vi "Speed From FFT (FPGA).vi"() -> ()   [LabVIEW 2013]
uses:
  <vilib>/Platform/TimedLoop/XDataNode/timing_clust.ctl
  <vilib>/Platform/TimedLoop/XDataNode/nitl_modes.ctl
  <vilib>/Platform/TimedLoop/XDataNode/wakeup.ctl
  <vilib>/rvi/FXPMathLib/FxpDiv/subVIs/nifxpmath_Div_SimConfig.ctl
  <vilib>/rvi/Emulation/niFpgaSctlEmulationGetInTimedLoop.vi
  <vilib>/rvi/Emulation/niFpgaEmulationReportErrorSimple.vi
  <vilib>/rvi/Emulation/niFpgaGetClockAttributes.vi
  <vilib>/rvi/eio/common/nirviEmuTemplateMethod_errors.vi
  <vilib>/rvi/Emulation/niFpgaCriticalErrorInLSC.vi
  <vilib>/rvi/Analysis/common/codeGenErrors/XNode/niFpgaXNodeCodeGenErrorHandle.vi
  <vilib>/rvi/Analysis/utilities/niFPGA Threshold Crossing Logic.vi
  <vilib>/rvi/FXPMathLib/FxpDiv/simVIs/DllFxpDivTemp_sub.vi
  <vilib>/rvi/interface/RandomDataEmulation/nirviRandomDataFPGAFIFO.vi
  <vilib>/rvi/interface/RandomDataEmulation/niFpgaRandomDataHandleErrors.vi
  <vilib>/rvi/DataTransferAndStorage/Container/Common/niFpgaContainerExecOnDevCompGetState.vi
  <vilib>/rvi/FIFO/Fifo_Resource/nirvififoEmulationWriteFpgaImpl.vi
  <vilib>/rvi/DataTransferAndStorage/Container/Common/niFpgaContainerGetUniqueNameForEmu.vi
  <vilib>/rvi/eio/common/nirviEmuReportErrorAndStop.vi
  <vilib>/eio/EIONode/EIONode.xnode
  <vilib>/rvi/Analysis/measure/period/templates/niFPGA Period Edge Direction.ctl
  <vilib>/rvi/FXPMathLib/FxpMul/XNode/nifxpmath_Multiplier.xnode
  <vilib>/rvi/FXPMathLib/FxpSub/XNode/nifxpmath_Sub.xnode
  <vilib>/rvi/Analysis/measure/butterworth/XNode/niFpgaButterworthFilter.xnode
  <vilib>/rvi/Analysis/measure/period/XNode/niFpgaAnalogPeriod.xnode
  <vilib>/Platform/TimedLoop/XDataNode/XDataNode.xnode
  <vilib>/rvi/FXPMathLib/FxpAdd/XNode/nifxpmath_Add.xnode
  <vilib>/rvi/FXPMathLib/FxpDiv/XNode/nifxpmath_Div.xnode
  <vilib>/rvi/DataTransferAndStorage/Container/XNode/niFpgaContainer.xnode
  <vilib>/rvi/interface/RandomDataEmulation/nirviRandomDataFpgaReadWriteTemplate.vi
  <vilib>/rvi/FIFO/Fifo_Resource/niFpgaFifoEmulationRefIn.vi
  <vilib>/rvi/FXPMathLib/sim/FxpSim.dll
  <vilib>/Platform/TimedLoop/XDataNode/XDNodeRunTimeDep.lvlib
panel:
  in  "under1enable":bool
  in  "thresh":fxp<+/-,24,7> format="%#_20g"
  in  "tresh calc":bool
  in  "PWM Duty":i32
  in  "PWM Period (ticks)":u32
  out "VerMult":fxp<+,20,20>
  in  "AveWidth":i32=7
  in  "CommSegs":i32=2
  in  "Hysteresis":fxp<+,10,6>
  in  "VoltCtrl":fxp<+/-,20,5>
  in  "PresCtrl":fxp<+/-,20,5>
  in  "PSenable":bool
  in  "stop":bool
  out "First":fxp<+/-,32,24>
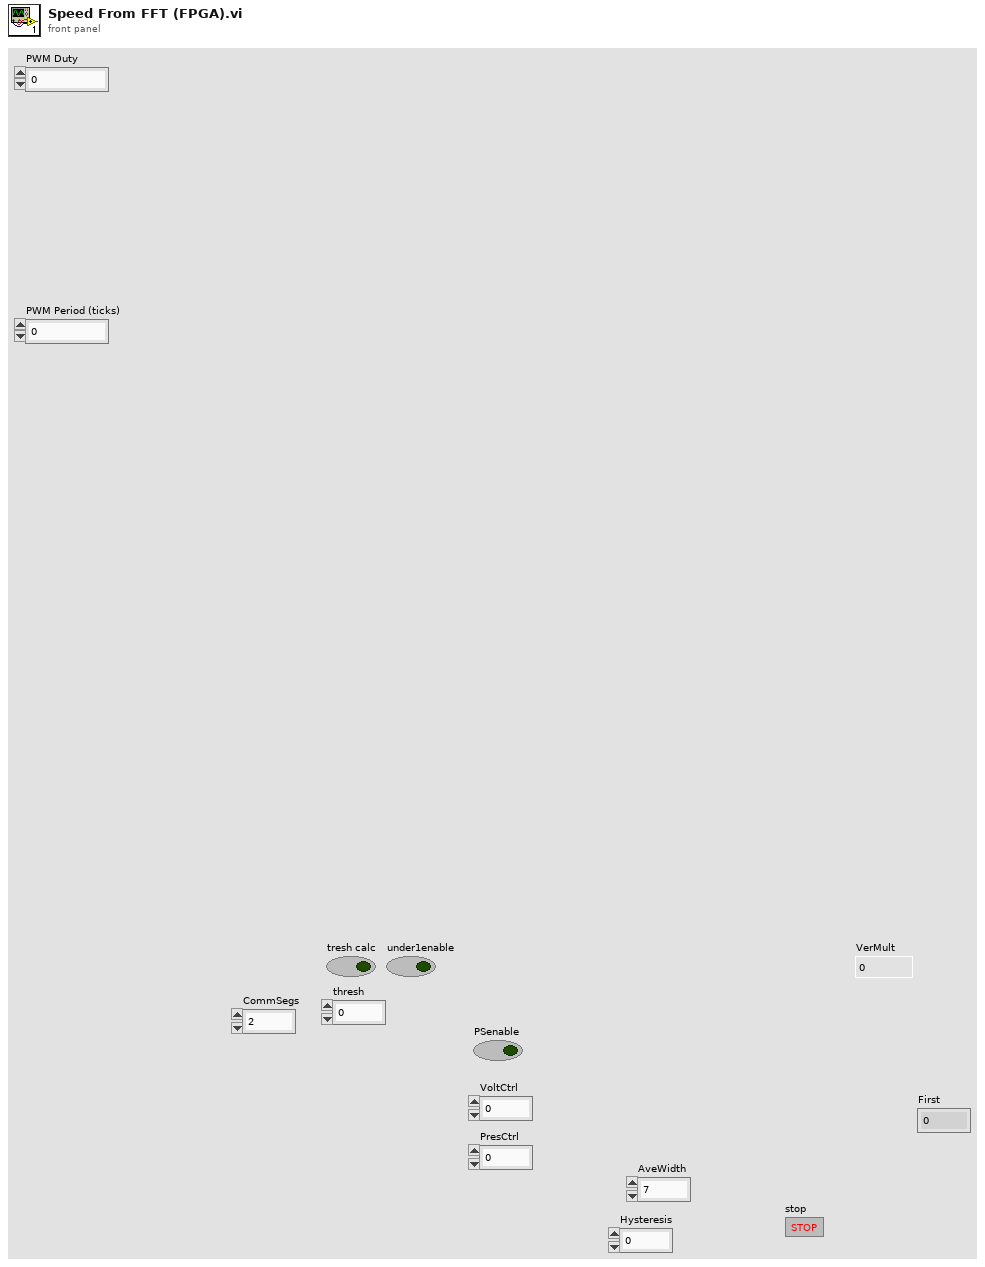
[diagram p1: front panel]
types:
  T1 = typedef "XDNodeRunTimeDep.lvlib/timing_clust.ctl" = cluster{"Expected End [f-1]":u64, "Actual End [f-1]":u64, "Finished Late? [f-1]":bool, "Expected End [i-1]":u64, "Actual End [i-1]":u64, "Finished Late? [i-1]":bool, "Expected Start [i]":u64, "Actual Start [i]":u64, "Expected Start [f]":u64, "Actual Start [f]":u64, "Source Name":string, "Structure Name":string, "Period":i64, "Deadline":i64, "Offset":i64, "Start":i64, "Priority":i32, "Timeout":i32, "Mode":T2, "Wakeup Reason":T3, "Error":errorcluster, "Source Type":string, "Secondary Source Type":string, "Global End Time":u64, "Global Start Time":u64, "Frame Duration":u64, "Iteration Duration":u64, "Assigned CPU":i32, "I/O Scan Engine Mode":u32}
  T2 = typedef "XDNodeRunTimeDep.lvlib/nitl_modes.ctl" = enum32{"No Change", "Process missed periods, maintain original phase", "Discard missed periods, maintain original phase", "Process missed periods, ignore original phase", "Discard missed periods, ignore original phase"}
  T3 = typedef "XDNodeRunTimeDep.lvlib/wakeup.ctl" = enum32{"Normal", "Aborted", "Asynchronous wakeup", "Timing source error", "Timed loop error", "Timeout"}
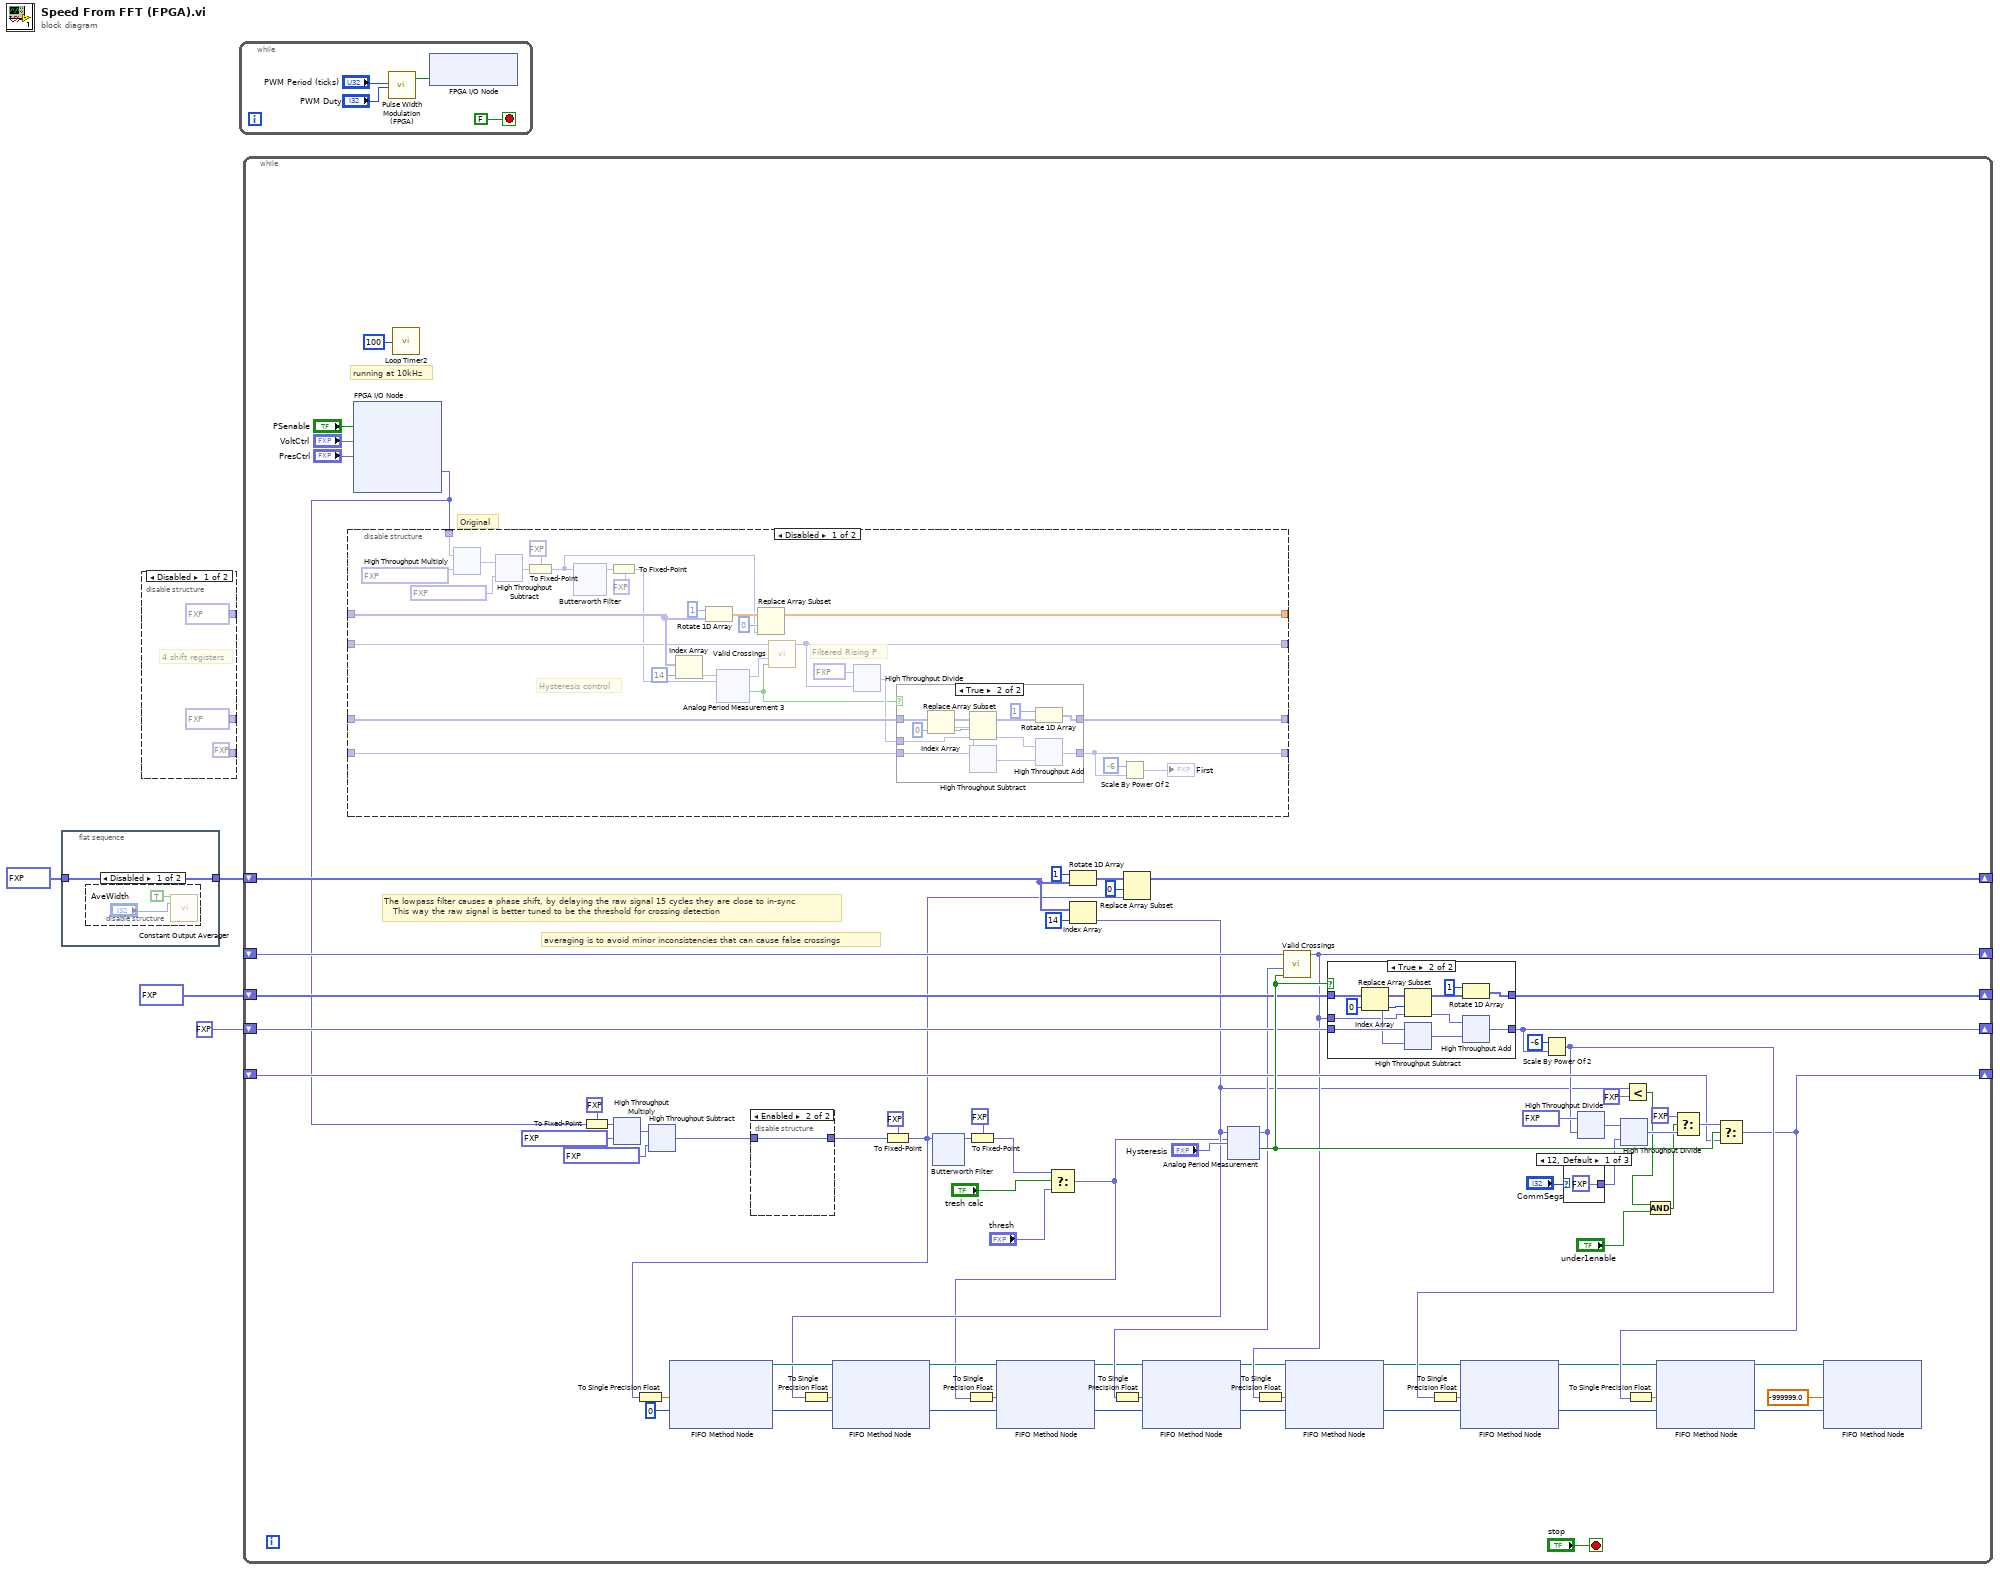
[diagram p0: block diagram]
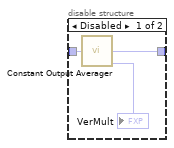
[diagram p4: hidden frame]
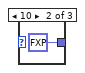
[diagram p6: hidden frame]
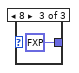
[diagram p7: hidden frame]
diagram:
  n1 = flat-sequence {
    tunnel: fxp<+/-,24,7>[] [0.0, 0.0, 0.0, 0.0, 0.0, 0.0, 0.0, 0.0, 0.0, 0.0, 0.0, 0.0, 0.0, 0.0, 0.0] -> [w5]
    tunnel: [w5] -> w1
    frame #0 {
      n2 = disable-structure shown="Disabled" {
        frame Disabled {
          n3 = call "Constant Output Averager.vi"("Init(T)/Run(F)"=TRUE, "AveWidth"="AveWidth") -> ()  [unwired: 12 in, 2 out]
        }
        frame Enabled {
        }
      }
    }
  }
  n4 = disable-structure shown="Disabled" {
    disable-tunnel: [fxp<+/-,24,6>[] [0.0, 0.0, 0.0, 0.0, 0.0, 0.0, 0.0, 0.0, 0.0, 0.0, 0.0, 0.0, 0.0, 0.0, 0.0] _] -> _
    disable-tunnel: [fxp<+/-,32,24> 0.0 ("mean") _] -> _
    disable-tunnel: [fxp<+/-,32,24>[] [0.0, 0.0, 0.0, 0.0, 0.0, 0.0, 0.0, 0.0, 0.0, 0.0, 0.0, 0.0, 0.0, 0.0, 0.0, 0.0, 0.0, 0.0, 0.0, 0.0, 0.0, 0.0, 0.0, 0.0, 0.0, 0.0, 0.0, 0.0, 0.0, 0.0, 0.0, 0.0, 0.0, 0.0, 0.0, 0.0, 0.0, 0.0, 0.0, 0.0, 0.0, 0.0, 0.0, 0.0, 0.0, 0.0, 0.0, 0.0, 0.0, 0.0, 0.0, 0.0, 0.0, 0.0, 0.0, 0.0, 0.0, 0.0, 0.0, 0.0, 0.0, 0.0, 0.0, 0.0] _] -> _
    frame Disabled {
      # "4 shift registers"
    }
    frame Enabled {
    }
  }
  n5 = while {
    stop <- FALSE stop-if-true
    n6 = call "Pulse Width Modulation (FPGA).vi"("PWM Period (Ticks)"="PWM Period (ticks)", "PWM Duty Cycle (Ticks)"="PWM Duty") -> ("PWM DO"=w14:bool)  [unwired: 14 in, 3 out]
    n7 = xnode "FPGA I/O Node"("RMC/DIO0"=w14) -> ()  [unwired: 1 in, 1 out]
  }
  n8 = while {
    shift-right: [w52] -> _
    shift-left: fxp<+/-,32,16> 0.0 ("mean") -> [w55]
    shift-right: [w51] -> _
    shift-left: fxp<+/-,32,16>[] [0.0, 0.0, 0.0, 0.0, 0.0, 0.0, 0.0, 0.0, 0.0, 0.0, 0.0, 0.0, 0.0, 0.0, 0.0, 0.0, 0.0, 0.0, 0.0, 0.0, 0.0, 0.0, 0.0, 0.0, 0.0, 0.0, 0.0, 0.0, 0.0, 0.0, 0.0, 0.0, 0.0, 0.0, 0.0, 0.0, 0.0, 0.0, 0.0, 0.0, 0.0, 0.0, 0.0, 0.0, 0.0, 0.0, 0.0, 0.0, 0.0, 0.0, 0.0, 0.0, 0.0, 0.0, 0.0, 0.0, 0.0, 0.0, 0.0, 0.0, 0.0, 0.0, 0.0, 0.0] -> [w49]
    shift-right: [w50] -> _
    shift-left: w1 -> [w56]
    shift-right: [w38] -> _
    shift-left: _ -> [w54]
    shift-right: [w35] -> _
    shift-left: _ -> [w53]
    stop <- "stop" stop-if-true
    w27 = 0 ("Timeout")
    # "averaging is to avoid minor inconsistencies that can cause false crossings"
    # "The lowpass filter causes a phase shift, by delaying the raw signal 15 cycles they are close to in-sync\n   This way the raw signal is better tuned to be the threshold for crossing detection"
    # "Original"
    # "running at 10kHz"
    n9 = xnode "FPGA I/O Node"("RMC/DIO1"="PSenable", "AO0"="VoltCtrl", "AO1"="PresCtrl") -> ("AI1"=w47:fxp<+/-,24,5>)  [unwired: 5 in, 6 out]
    n10 = disable-structure shown="Disabled" {
      disable-tunnel: _ -> [w301 _]
      disable-tunnel: [w300 _] -> _
      disable-tunnel: _ -> [w296 _]
      disable-tunnel: [w294 _] -> _
      disable-tunnel: [w293 _] -> _
      disable-tunnel: _ -> [w292 _]
      disable-tunnel: _ -> [w291 _]
      disable-tunnel: [w290 _] -> _
      disable-tunnel: w47 -> [w287 _]
      frame Disabled {
        # "Hysteresis control"
        # "Filtered Rising P"
        n11 = xnode ("High Throughput Multiply")("x"=w287, "y"=fxp<+/-,20,7> 24.0384521484375 ("Volt")) -> ("x*y"=w308:fxp<+/-,44,12>)
        n12 = xnode "High Throughput Subtract"("x"=w308, "y"=fxp<+/-,20,7> 60.09619140625 ("Volt")) -> ("x-y"=w284:fxp<+/-,24,7>)
        n13 = To Fixed-Point(fixed-point type=fxp<+,24,5> 0.0 ("AI4"), number=w284) -> (fixed-point=w297:fxp<+,24,5>)
        n14 = xnode "Butterworth Filter"("input data"=w297) -> ("output data"=w299:fxp<+/-,29,10>)  [unwired: 2 in]
        n15 = To Fixed-Point(fixed-point type=fxp<+/-,24,6> 0.0 ("threshold level"), number=w299) -> (fixed-point=w285:fxp<+/-,24,6>)
        n16 = Index Array(array=w301, index=14) -> (element=w279)
        n17 = Rotate 1D Array(1:w301, 2:1 ("n")) -> (0:w303:ext[])
        n18 = xnode ("Analog Period Measurement 3")("input data"=w279, "threshold level"=w285) -> ("hysteresis"=w282:fxp<+,23,5>, "period (samples)"=w281:fxp<+,32,16>, "output valid"=w288:bool)  [unwired: 2 in, 2 out]
        n19 = Replace Array Subset(array=w303, new element=w297, index=0) -> (w300:ext[])
        n20 = call "Valid Crossings.vi"("Input Valid?"=w288, "Value In"=w281, "Reference"=w296) -> ("Value Out"=w290:fxp<+,32,16>)  [unwired: 8 in]
        n21 = xnode "High Throughput Divide"("x"=fxp<+,32,20> 75000.0, "y"=w290) -> ("x/y"=w289:fxp<+,36,36>)
        n22 = case shown="True" w288 {
          tunnel: w291 -> [w310 w317]
          tunnel: [w310 w319] -> w293
          tunnel: w292 -> [w309 w315]
          tunnel: [w309 w312] -> w294
          tunnel: w289 -> [_ w311]
          frame False {
          }
          frame True {
            w316 = 0 ("index")
            n23 = Index Array(array=w317, index=w316) -> (element=w314)
            n24 = Replace Array Subset(array=w317, new element=w311, index=w316) -> (w320:fxp<+,36,36>[])
            n25 = xnode "High Throughput Subtract"("x"=w315, "y"=w314) -> ("x-y"=w313:fxp<+/-,32,24>)
            n26 = Rotate 1D Array(1:w320, 2:1 ("n")) -> (0:w319:fxp<+,36,36>[])
            n27 = xnode "High Throughput Add"("x"=w311, "y"=w313) -> ("x+y"=w312:fxp<+/-,32,24>)
          }
        }
        n28 = Scale By Power Of 2(n=i16 -6, x=w294) -> (x*2^n=→"First":fxp<+/-,32,24>)
      }
      frame Enabled {
      }
    }
    n29 = call "Loop Timer2"("Count(uSec)"=u32 100 ("Count(Ticks)")) -> ()  [unwired: 1 out]
    n30 = To Fixed-Point(fixed-point type=fxp<+,24,5> 0.0 ("AI4"), number=w47) -> (fixed-point=w46:fxp<+,24,5>)
    n31 = xnode ("High Throughput Multiply")("x"=w46, "y"=fxp<+/-,20,7> 24.0384521484375 ("Volt")) -> ("x*y"=w58:fxp<+/-,44,12>)
    n32 = xnode "High Throughput Subtract"("x"=w58, "y"=fxp<+/-,20,7> 60.09619140625 ("Volt")) -> ("x-y"=w26:fxp<+/-,24,7>)
    n33 = disable-structure shown="Enabled" {
      disable-tunnel: w26 -> [w85 w86]
      disable-tunnel: [w84 w86] -> w25
      frame Disabled {
        n34 = call "Constant Output Averager.vi"("Input"=w85) -> ("Output"=w84:fxp<+/-,62,46>, "VerMult"=→"VerMult":fxp<+,20,20>)  [unwired: 13 in]
      }
      frame Enabled {
      }
    }
    n35 = To Fixed-Point(fixed-point type=fxp<+/-,24,7> 0.0 ("x-y"), number=w25) -> (fixed-point=w24:fxp<+/-,24,7>)
    n36 = To Single Precision Float(number=w24) -> (single precision float=w40:sgl)
    n37 = xnode ("FIFO Method Node")("Element"=w40, "Timeout"=w27) -> ("FIFO Out"=w34:refnum<k21>)  [unwired: 1 in, 1 out]
    n38 = xnode "Butterworth Filter"("input data"=w24) -> ("output data"=w65:fxp<+/-,28,11>)  [unwired: 2 in]
    n39 = To Fixed-Point(fixed-point type=fxp<+/-,24,7> 0.0 ("threshold level"), number=w65) -> (fixed-point=w21:fxp<+/-,24,7>)
    n40 = Select(t=w21, s="tresh calc", f="thresh") -> (s? t:f=w18:fxp<+/-,24,7>)
    n41 = To Single Precision Float(number=w18) -> (single precision float=w42:sgl)
    n42 = Rotate 1D Array(1:w56, 2:1 ("n")) -> (0:w71:fxp<+/-,24,7>[])
    n43 = Index Array(array=w56, index=14) -> (element=w22:fxp<+/-,24,7>)
    n44 = To Single Precision Float(number=w22) -> (single precision float=w41:sgl)
    n45 = xnode ("FIFO Method Node")("Element"=w41, "Timeout"=w27, "FIFO In"=w34) -> ("FIFO Out"=w33:refnum<k21>)  [unwired: 1 out]
    n46 = xnode ("FIFO Method Node")("Element"=w42, "Timeout"=w27, "FIFO In"=w33) -> ("FIFO Out"=w32:refnum<k21>)  [unwired: 1 out]
    n47 = Replace Array Subset(array=w71, new element=w24, index=0) -> (w50:fxp<+/-,24,7>[])
    n48 = xnode ("Analog Period Measurement")("input data"=w22, "threshold level"=w18, "hysteresis"="Hysteresis") -> ("period (samples)"=w39:fxp<+,32,16>, "output valid"=w76:bool)  [unwired: 2 in, 2 out]
    n49 = To Single Precision Float(number=w39) -> (single precision float=w43:sgl)
    n50 = xnode ("FIFO Method Node")("Element"=w43, "Timeout"=w27, "FIFO In"=w32) -> ("FIFO Out"=w31:refnum<k21>)  [unwired: 1 out]
    n51 = call "Valid Crossings.vi"("Input Valid?"=w76, "Value In"=w39, "Reference"=w54) -> ("Value Out"=w38:fxp<+,32,16>)  [unwired: 8 in]
    n52 = To Single Precision Float(number=w38) -> (single precision float=w44:sgl)
    n53 = xnode ("FIFO Method Node")("Element"=w44, "Timeout"=w27, "FIFO In"=w31) -> ("FIFO Out"=w30:refnum<k21>)  [unwired: 1 out]
    n54 = case shown="True" w76 {
      tunnel: w49 -> [w88 w95]
      tunnel: [w88 w97] -> w51
      tunnel: w55 -> [w87 w93]
      tunnel: [w87 w90] -> w52
      tunnel: w38 -> [_ w89]
      frame False {
      }
      frame True {
        w94 = 0 ("index")
        n55 = Index Array(array=w95, index=w94) -> (element=w92:fxp<+/-,32,16>)
        n56 = Replace Array Subset(array=w95, new element=w89, index=w94) -> (w98:fxp<+/-,32,16>[])
        n57 = xnode "High Throughput Subtract"("x"=w93, "y"=w92) -> ("x-y"=w91:fxp<+/-,32,16>)
        n58 = Rotate 1D Array(1:w98, 2:1 ("n")) -> (0:w97:fxp<+/-,32,16>[])
        n59 = xnode ("High Throughput Add")("x"=w89, "y"=w91) -> ("x+y"=w90:fxp<+/-,32,16>)
      }
    }
    n60 = Scale By Power Of 2(n=i16 -6, x=w52) -> (x*2^n=w36:fxp<+/-,32,16>)
    n61 = To Single Precision Float(number=w36) -> (single precision float=w37:sgl)
    n62 = xnode ("FIFO Method Node")("Element"=w37, "Timeout"=w27, "FIFO In"=w30) -> ("FIFO Out"=w29:refnum<k21>)  [unwired: 1 out]
    n63 = case shown="12, Default" "CommSegs" {
      tunnel: [fxp<+,4,4> 1.0 ("y") fxp<+,4,4> 5.0 ("y") fxp<+,4,4> 4.0 ("y")] -> w68
      frame 12, Default {
      }
      frame 10 {
      }
      frame 8 {
      }
    }
    n64 = xnode "High Throughput Divide"("x"=fxp<+,32,20> 300000.0, "y"=w36) -> ("x/y"=w64:fxp<+/-,37,37>)
    n65 = xnode "High Throughput Divide"("x"=w64, "y"=w68) -> ("x/y"=w69:fxp<+/-,37,37>)
    n66 = Less?(x=w22, y=fxp<+,14,6> 1.0) -> (x < y?=w17:bool)
    n67 = And(x=w17, y="under1enable") -> (x .and. y?=w16:bool)
    n68 = Select(t=fxp<+,36,36> 0.0, s=w16, f=w69) -> (s? t:f=w66:fxp<+/-,37,37>)
    n69 = Select(t=w66, s=w76, f=w53) -> (s? t:f=w35:fxp<+/-,37,37>)
    n70 = To Single Precision Float(number=w35) -> (single precision float=w45:sgl)
    n71 = xnode ("FIFO Method Node")("Element"=w45, "Timeout"=w27, "FIFO In"=w29) -> ("FIFO Out"=w28:refnum<k21>)  [unwired: 1 out]
    n72 = xnode ("FIFO Method Node")("Element"=sgl -999999.0, "Timeout"=w27, "FIFO In"=w28) -> ()  [unwired: 2 out]
  }
